vi "Parse DB - 1553 - Get BC Config.vi"(0 "channel config handle":u32, 11 "error in (no error)":errorcluster) -> (4 "channel config handle out":u32, 6 "Bus_Controller":T1, 8 "Xfer Count != Buffer Count":bool, 15 "error out":errorcluster)   [LabVIEW 2013, in "AIT 1553 Custom Device.lvlib"]
uses:
  AIT 1553 Custom Device.lvlib
  Controls/1553_Bus_Controller.ctl
  Controls/1553_BC_Message.ctl
  Controls/1553 Param.ctl
  Controls/1553_Acyclic_Frame.ctl
  <userlib>/MIL-STD-1553/Owl1553.lvlib
panel:
  out "description":string
  out "Xfer count":u32
  out "buffer count":u32
  out "BC Initial Buffer Data":u16[][](array[numeric]) format="%.0x"
  out "BC Sizes":u32[](array[numeric])
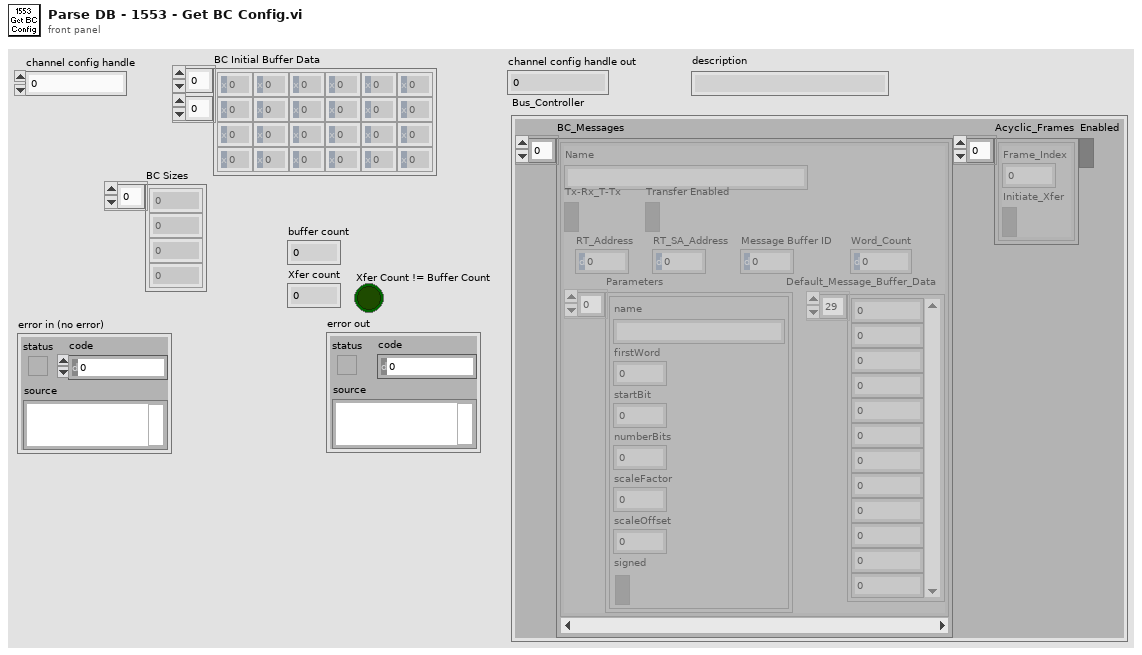
[diagram p1: front panel]
types:
  T1 = typedef "AIT 1553 Custom Device.lvlib/1553_Bus_Controller.ctl" = cluster{"BC_Messages":T2[], "Acyclic_Frames":T4[], "Enabled":bool}
  T2 = typedef "AIT 1553 Custom Device.lvlib/1553_BC_Message.ctl" = cluster{"Name":string, "Tx-Rx_T-Tx":bool, "RT_Address":u8, "RT_SA_Address":u8, "Parameters":T3[], "Transfer Enabled":bool, "Message Buffer ID":u16, "Default_Message_Buffer_Data":u16[], "Word_Count":u8}
  T3 = typedef "AIT 1553 Custom Device.lvlib/1553 Param.ctl" = cluster{"name":string, "firstWord":i32, "startBit":i32, "numberBits":i32, "scaleFactor":dbl, "scaleOffset":dbl, "signed":bool}
  T4 = typedef "AIT 1553 Custom Device.lvlib/1553_Acyclic_Frame.ctl" = cluster{"Frame_Index":u8, "Initiate_Xfer":bool}
  T5 = enum16{"OWL1553_BCRT", "OWL1553_RTBC", "OWL1553_RTRT", "OWL1553_FRONT_HALF", "OWL1553_BACK_HALF", "OWL1553_MSG_ERROR"}
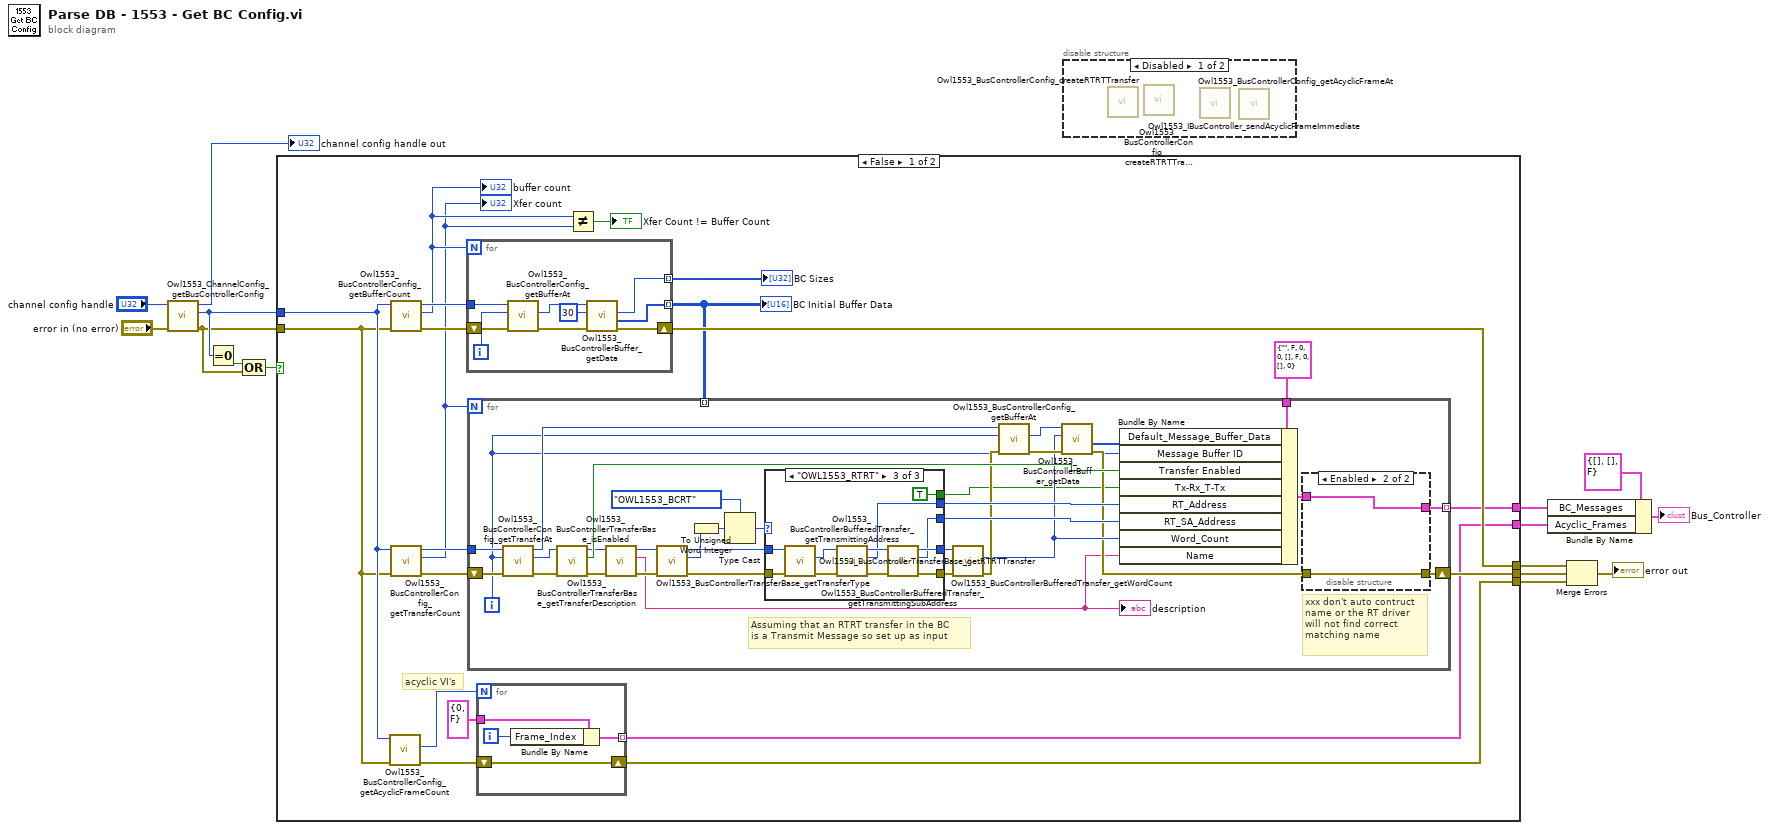
[diagram p0: block diagram]
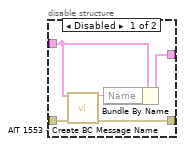
[diagram p2: hidden frame]
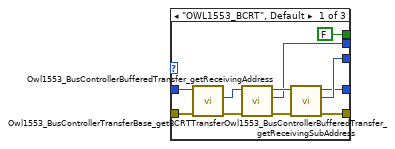
[diagram p3: hidden frame]
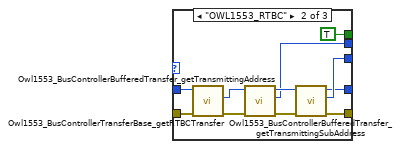
[diagram p4: hidden frame]
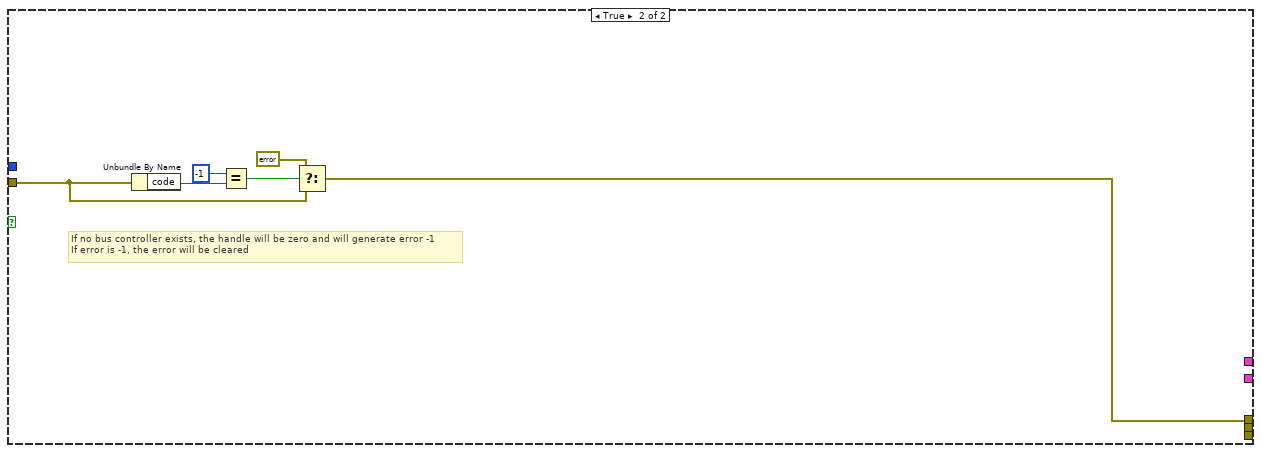
[diagram p5: hidden frame]
diagram:
  n1 = call <userlib>:"Owl1553_ChannelConfig_getBusControllerConfig.vi"("error in (no error)"="error in (no error)", "channel config handle"="channel config handle") -> ("error out"=w3:errorcluster, "bus controller config handle"=w4:u32, "channel config handle"=→"channel config handle out":u32)  [unwired: 7 in]
  n2 = Equal To 0?(x=w4) -> (x = 0?=w2:bool)
  n3 = Compound Arithmetic op=OR(w2, w3) -> (w1:bool)
  n4 = case shown="False" w1 {
    tunnel: [w27 _] -> w13
    tunnel: [w26 w122] -> w12
    tunnel: [w24 _] -> w10
    tunnel: w4 -> [w22 _]
    tunnel: w3 -> [w21 w123]
    tunnel: [w17 _] -> w7
    tunnel: [w16 _] -> w6
    frame False {
      # "acyclic VI's"
      n5 = call <userlib>:"Owl1553_BusControllerConfig_getAcyclicFrameCount.vi"("error in (no error)"=w21, "bus controller config handle"=w22) -> ("error out"=w19:errorcluster, "acyclic frame count"=w20:u32)  [unwired: 7 in, 1 out]
      n6 = call <userlib>:"Owl1553_BusControllerConfig_getBufferCount.vi"("error in (no error)"=w21, "bus controller config handle"=w22) -> ("error out"=w34:errorcluster, "buffer count"=w29:u32, "bus controller config handle"=w33:u32)  [unwired: 7 in]
      "buffer count" <- w29
      n7 = call <userlib>:"Owl1553_BusControllerConfig_getTransferCount.vi"("error in (no error)"=w21, "bus controller config handle"=w22) -> ("error out"=w32:errorcluster, "transfer count"=w23:u32, "bus controller config handle"=w31:u32)  [unwired: 7 in]
      "Xfer count" <- w23
      n8 = for {
        N: w29 -> [_]
        tunnel: w33 -> [w121]
        tunnel: [w113] -> w25 mode=indexing
        tunnel: [w118] -> w35 mode=indexing
        shift-right: [w117] -> w26
        shift-left: w34 -> [w120]
        i -> [w119]
        n9 = call <userlib>:"Owl1553_BusControllerConfig_getBufferAt.vi"("error in (no error)"=w120, "index"=w119, "bus controller config handle"=w121) -> ("error out"=w116:errorcluster, "buffer handle"=w115:u32)  [unwired: 6 in, 1 out]
        n10 = call <userlib>:"Owl1553_BusControllerBuffer_getData.vi"("error in (no error)"=w116, "buffer size"=u32 30, "bus controller buffer handle"=w115) -> ("error out"=w117:errorcluster, "data"=w113:u16[], "buffer size out"=w118:u32)  [unwired: 5 in, 1 out]
      }
      "BC Initial Buffer Data" <- w25
      "BC Sizes" <- w35
      n11 = for {
        N: w23 -> [_]
        tunnel: w31 -> [w67]
        tunnel: T2 {"Name"="", "Tx-Rx_T-Tx"=FALSE, "RT_Address"=0, "RT_SA_Address"=0, "Parameters"=[], "Transfer Enabled"=FALSE, "Message Buffer ID"=0, "Default_Message_Buffer_Data"=[], "Word_Count"=0} ("BC_Message") -> [w64]
        tunnel: [w54] -> w24 mode=indexing
        tunnel: w25 -> [_] mode=indexing
        shift-right: [w60] -> w27
        shift-left: w32 -> [w72]
        i -> [w46]
        # "Assuming that an RTRT transfer in the BC\nis a Transmit Message so set up as input"
        # "xxx don't auto contruct\nname or the RT driver\nwill not find correct\nmatching name"
        n12 = call <userlib>:"Owl1553_BusControllerConfig_getTransferAt.vi"("error in (no error)"=w72, "index"=w46, "bus controller config handle"=w67) -> ("error out"=w68:errorcluster, "transfer base handle"=w65:u32, "bus controller config handle"=w47:u32)  [unwired: 6 in]
        n13 = call <userlib>:"Owl1553_BusControllerTransferBase_isEnabled.vi"("error in (no error)"=w68, "transferbase handle"=w65) -> ("error out"=w57:errorcluster, "enabled"=w59:bool, "transferbase handle"=w58:u32)  [unwired: 6 in]
        n14 = call "Owl1553_BusControllerTransferBase_getTransferDescription.vi"("error in (no error)"=w57, "transferbase handle"=w58) -> ("error out"=w56:errorcluster, "transferdescription"=w44:string, "transferbase handle"=w55:u32)  [unwired: 6 in]
        "description" <- w44
        n15 = call <userlib>:"Owl1553_BusControllerTransferBase_getTransferType.vi"("error in (no error)"=w56, "transferbase handle"=w55) -> ("error out"=w70:errorcluster, "transfer type"=w42:i32, "transferbase handle"=w66:u32)  [unwired: 6 in]
        n16 = To Unsigned Word Integer(number=w42) -> (unsigned 16bit integer=w45:u16)
        n17 = Type Cast(type=T5."OWL1553_BCRT" ("Owl1553TransferMessageType"), x=w45) -> (*(type *) &x=w41:T5)
        n18 = case shown="\"OWL1553_RTRT\"" w41 {
          tunnel: w70 -> [w90 w101 w111]
          tunnel: [w84 w95 w104] -> w71
          tunnel: [w83 w96 w103] -> w69
          tunnel: w66 -> [w89 w100 w112]
          tunnel: [w86 w94 w106] -> w62
          tunnel: [w85 w97 w102] -> w63
          tunnel: [FALSE ("Initiate_Xfer") TRUE ("Initiate_Xfer") TRUE ("Initiate_Xfer")] -> w40
          frame "OWL1553_BCRT", Default {
            n19 = call <userlib>:"Owl1553_BusControllerTransferBase_getBCRTTransfer.vi"("error in (no error)"=w90, "transferbase handle"=w89) -> ("error out"=w82:errorcluster, "bcrt transfer handle"=w81:u32)  [unwired: 6 in, 1 out]
            n20 = call <userlib>:"Owl1553_BusControllerBufferedTransfer_getReceivingAddress.vi"("error in (no error)"=w82, "buffered transfer handle"=w81) -> ("error out"=w88:errorcluster, "remote terminal address"=w86:u8, "buffered transfer handle"=w87:u32)  [unwired: 6 in]
            n21 = call <userlib>:"Owl1553_BusControllerBufferedTransfer_getReceivingSubAddress.vi"("error in (no error)"=w88, "buffered transfer handle"=w87) -> ("error out"=w84:errorcluster, "remote terminal address"=w85:u8, "buffered transfer handle"=w83:u32)  [unwired: 6 in]
          }
          frame "OWL1553_RTBC" {
            n22 = call <userlib>:"Owl1553_BusControllerTransferBase_getRTBCTransfer.vi"("error in (no error)"=w101, "transferbase handle"=w100) -> ("error out"=w92:errorcluster, "rtbc transfer handle"=w93:u32)  [unwired: 6 in, 1 out]
            n23 = call <userlib>:"Owl1553_BusControllerBufferedTransfer_getTransmittingAddress.vi"("error in (no error)"=w92, "buffered transfer handle"=w93) -> ("error out"=w99:errorcluster, "remote terminal address"=w94:u8, "buffered transfer handle"=w98:u32)  [unwired: 6 in]
            n24 = call <userlib>:"Owl1553_BusControllerBufferedTransfer_getTransmittingSubAddress.vi"("error in (no error)"=w99, "buffered transfer handle"=w98) -> ("error out"=w95:errorcluster, "remote terminal sub-address"=w97:u8, "buffered transfer handle"=w96:u32)  [unwired: 6 in]
          }
          frame "OWL1553_RTRT" {
            n25 = call <userlib>:"Owl1553_BusControllerTransferBase_getRTRTTransfer.vi"("error in (no error)"=w111, "transferbase handle"=w112) -> ("error out"=w107:errorcluster, "rtrt transfer handle"=w108:u32)  [unwired: 6 in, 1 out]
            n26 = call <userlib>:"Owl1553_BusControllerBufferedTransfer_getTransmittingAddress.vi"("error in (no error)"=w107, "buffered transfer handle"=w108) -> ("error out"=w105:errorcluster, "remote terminal address"=w106:u8, "buffered transfer handle"=w109:u32)  [unwired: 6 in]
            n27 = call <userlib>:"Owl1553_BusControllerBufferedTransfer_getTransmittingSubAddress.vi"("error in (no error)"=w105, "buffered transfer handle"=w109) -> ("error out"=w104:errorcluster, "remote terminal sub-address"=w102:u8, "buffered transfer handle"=w103:u32)  [unwired: 6 in]
          }
        }
        n28 = call <userlib>:"Owl1553_BusControllerBufferedTransfer_getWordCount.vi"("error in (no error)"=w71, "buffered transfer handle"=w69) -> ("error out"=w51:errorcluster, "word count"=w50:u8)  [unwired: 6 in, 1 out]
        n29 = call <userlib>:"Owl1553_BusControllerConfig_getBufferAt.vi"("error in (no error)"=w51, "index"=w46, "bus controller config handle"=w47) -> ("error out"=w52:errorcluster, "buffer handle"=w53:u32)  [unwired: 6 in, 1 out]
        n30 = call <userlib>:"Owl1553_BusControllerBuffer_getData.vi"("error in (no error)"=w52, "buffer size"=w50, "bus controller buffer handle"=w53) -> ("error out"=w48:errorcluster, "data"=w49:u16[])  [unwired: 5 in, 2 out]
        n31 = Bundle By Name(cluster=w64, "Default_Message_Buffer_Data"=w49, "Message Buffer ID"=w46, "Transfer Enabled"=w59, "Tx-Rx_T-Tx"=w40, "RT_Address"=w62, "RT_SA_Address"=w63, "Word_Count"=w50, "Name"=w44) -> (w61:T2)
        n32 = disable-structure shown="Enabled" {
          disable-tunnel: w61 -> [w77 w79]
          disable-tunnel: w48 -> [w76 w78]
          disable-tunnel: [w75 w78] -> w60
          disable-tunnel: [w73 w79] -> w54
          frame Disabled {
            n33 = call "AIT 1553 - Create BC Message Name.vi"("BC_Message"=w77, "error in (no error)"=w76) -> ("Message Name"=w74:string, "error out"=w75:errorcluster)  [unwired: 12 in]
            n34 = Bundle By Name(cluster=w77, "Name"=w74) -> (w73:T2)
          }
          frame Enabled {
          }
        }
      }
      n35 = for {
        N: w20 -> [_]
        tunnel: T4 {"Frame_Index"=0, "Initiate_Xfer"=FALSE} ("Acyclic_Frame") -> [w39]
        tunnel: [w36] -> w16 mode=indexing
        shift-right: [w37] -> w17
        shift-left: w19 -> [w37]
        i -> [w38]
        n36 = Bundle By Name(cluster=w39, "Frame_Index"=w38) -> (w36:T4)
      }
      n37 = Not Equal?(x=w29, y=w23) -> (x != y?=→"Xfer Count != Buffer Count":bool)
    }
    frame True {
      # "If no bus controller exists, the handle will be zero and will generate error -1\nIf error is -1, the error will be cleared"
      n38 = Unbundle By Name(w123) -> ("code"=w127:i32)
      n39 = Equal?(x=-1, y=w127) -> (x = y?=w125:bool)
      n40 = Select(t=errorcluster {"status"=FALSE, "code"=0, "source"=""} ("error out"), s=w125, f=w123) -> (s? t:f=w122:errorcluster)
    }
  }
  n41 = disable-structure shown="Disabled" {
    frame Disabled {
      # "RT to RT"
      n42 = call <userlib>:"Owl1553_BusControllerConfig_createRTRTTransfer.vi"() -> ()  [unwired: 8 in, 4 out]
      n43 = call <userlib>:"Owl1553_BusControllerConfig_createRTRTTransferWithDescription.vi"() -> ()  [unwired: 11 in, 5 out]
      n44 = call <userlib>:"Owl1553_BusControllerConfig_getAcyclicFrameAt.vi"() -> ()  [unwired: 9 in, 3 out]
      n45 = call <userlib>:"Owl1553_IBusController_sendAcyclicFrameImmediate.vi"() -> ()  [unwired: 10 in, 2 out]
    }
    frame Enabled {
    }
  }
  n46 = Bundle By Name(cluster=T1 {"BC_Messages"=[], "Acyclic_Frames"=[], "Enabled"=FALSE} ("Bus_Controller"), "BC_Messages"=w10, "Acyclic_Frames"=w6) -> (→"Bus_Controller":T1)
  n47 = Merge Errors(w12, w13, w7) -> (→"error out":errorcluster)
